vi "LVClass_SlopesPostProcessList AddProcessor_NeighboorExtension&ShutOfBoundaries.vi"(0 "SlopesPostProcessorList.lvclass":refnum<class "SlopesPostProcessorList.lvclass">, 2 "Neighborhood Extension":bool, 3 "ShutOfBoundaries":u32, 5 "error in (no error)":errorcluster) -> (14 "SlopesPostProcessorList out":refnum<class "SlopesPostProcessorList.lvclass">, 19 "error out":errorcluster)   [LabVIEW 2020, in "SlopesPostProcessorList.lvclass"]
uses:
  SlopesPostProcessorList.lvclass
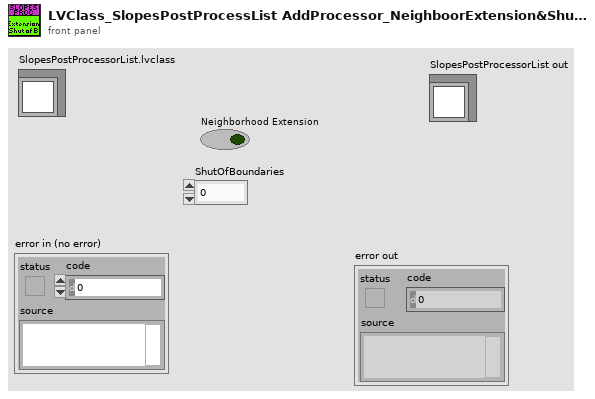
[diagram p1: front panel]
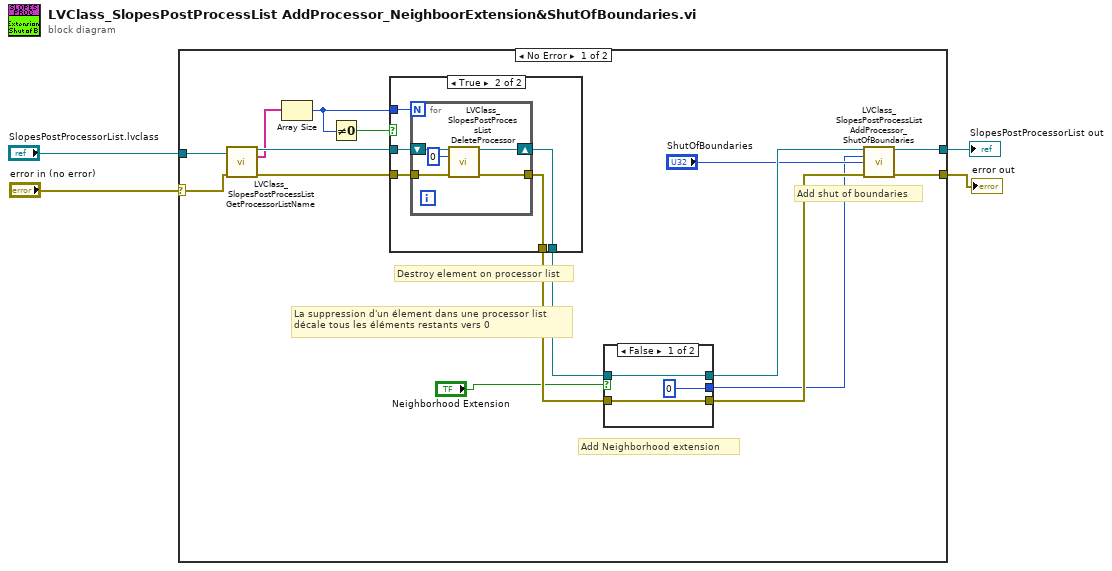
[diagram p0: block diagram]
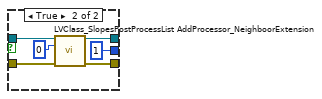
[diagram p3: hidden frame]
diagram:
  n1 = case shown="No Error" "error in (no error)" {
    selector: "error in (no error)" -> [w9 w42]
    tunnel: "SlopesPostProcessorList.lvclass" -> [w20 w43]
    tunnel: [w12 w43] -> w3
    tunnel: [w11 w42] -> w2
    frame No Error {
      # "La suppression d'un élement dans une processor list \ndécale tous les éléments restants vers 0"
      # "Add shut of boundaries"
      # "Add Neighborhood extension"
      # "Destroy element on processor list"
      n2 = call "LVClass_SlopesPostProcessList GetProcessorListName.vi"("SlopesPostProcessorList in"=w20, "error in (no error)"=w9) -> ("SlopesPostProcessorList out"=w19:refnum<class "SlopesPostProcessorList.lvclass">, "name"=w5:string[], "error out"=w18:errorcluster)  [unwired: 11 in]
      n3 = Array Size(array=w5) -> (size(s)=w6:i32)
      n4 = Not Equal To 0?(x=w6) -> (x != 0?=w7:bool)
      n5 = case shown="True" w7 {
        tunnel: w6 -> [_ w27]
        tunnel: w19 -> [w22 w26]
        tunnel: w18 -> [w21 w25]
        tunnel: [w22 w24] -> w17
        tunnel: [w21 w23] -> w16
        frame False {
        }
        frame True {
          n6 = for {
            N: w27 -> [_]
            tunnel: w25 -> [w31]
            tunnel: [w29] -> w23
            shift-right: [w30] -> w24
            shift-left: w26 -> [w32]
            n7 = call "LVClass_SlopesPostProcessList DeleteProcessor.vi"("SlopesPostProcessorList in"=w32, "Position"=0, "error in (no error)"=w31) -> ("SlopesPostProcessorList out"=w30:refnum<class "SlopesPostProcessorList.lvclass">, "error out"=w29:errorcluster)  [unwired: 11 in]
          }
        }
      }
      n8 = case shown="False" "Neighborhood Extension" {
        tunnel: w17 -> [w35 w41]
        tunnel: w16 -> [w34 w40]
        tunnel: [w35 w38] -> w15
        tunnel: [w34 w37] -> w13
        tunnel: [u32 0 ("ShutOfBoundaries") u32 1 ("ShutOfBoundaries")] -> w8
        frame False {
        }
        frame True {
          n9 = call "LVClass_SlopesPostProcessList AddProcessor_NeighboorExtension.vi"("SlopesPostProcessorList in"=w41, "Position"=0, "error in (no error)"=w40) -> ("SlopesPostProcessorList out"=w38:refnum<class "SlopesPostProcessorList.lvclass">, "error out"=w37:errorcluster)  [unwired: 11 in]
        }
      }
      n10 = call "LVClass_SlopesPostProcessList AddProcessor_ShutOfBoundaries.vi"("SlopesPostProcessorList in"=w15, "Position"=w8, "ShutOfBoundaries"="ShutOfBoundaries", "error in (no error)"=w13) -> ("SlopesPostProcessorList out"=w12:refnum<class "SlopesPostProcessorList.lvclass">, "error out"=w11:errorcluster)  [unwired: 10 in]
    }
    frame Error {
    }
  }
  "error out" <- w2
  "SlopesPostProcessorList out" <- w3
